vi "parse load from string.vi"(8 "error in":errorcluster, 11 "message data":string) -> (0 "error out":errorcluster, 2 "targets to load":string[](array[string]), 3 "system data":string)   [LabVIEW 2013, in "module execution process.lvlib"]
uses:
  module execution process.lvlib
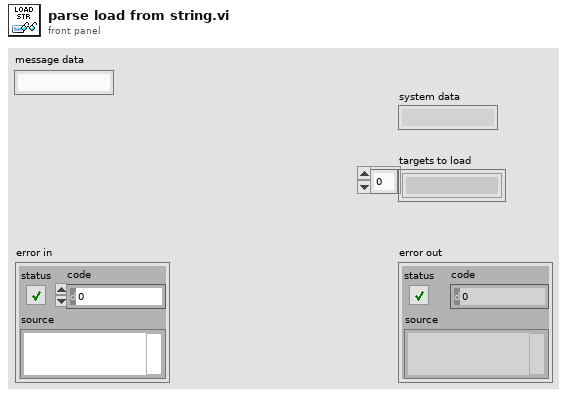
[diagram p1: front panel]
types:
  T1 = cluster{"system data":string, "targets to load":string[]}
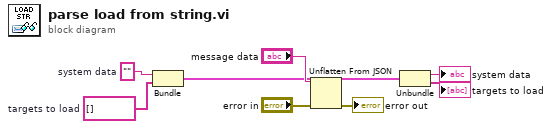
[diagram p0: block diagram]
diagram:
  w5 = string[] []  # targets to load
  w6 = ""  # system data
  n1 = Bundle("system data"=w6, "targets to load"=w5) -> (w4:T1)  [unwired: 1 in]
  n2 = Unflatten From JSON(JSON string="message data", type and defaults=w4, error in (no error)="error in") -> (value=w3:T1, error out=→"error out":errorcluster)  [unwired: 4 in]
  n3 = Unbundle(w3) -> ("system data"=→"system data":string, "targets to load"=→"targets to load":string[])
